vi "swabian_buffer_to_photons.vi"(0 "buffer":u64[](array[numeric]), 4 "Leftovers_in":T1, 5 "error in (no error)":errorcluster, 6 "sync_channel":i32, 8 "sync_period_ps":u64, 10 "first_batch":i32, 12 "first_sync_stamp":u64) -> (14 "output_buffer":u64[](array[numeric]), 15 "first_sync_stamp_out":u64, 18 "Leftovers_out":T1, 19 "error out":errorcluster)   [LabVIEW 2018]
uses:
  swabian_lib.dll
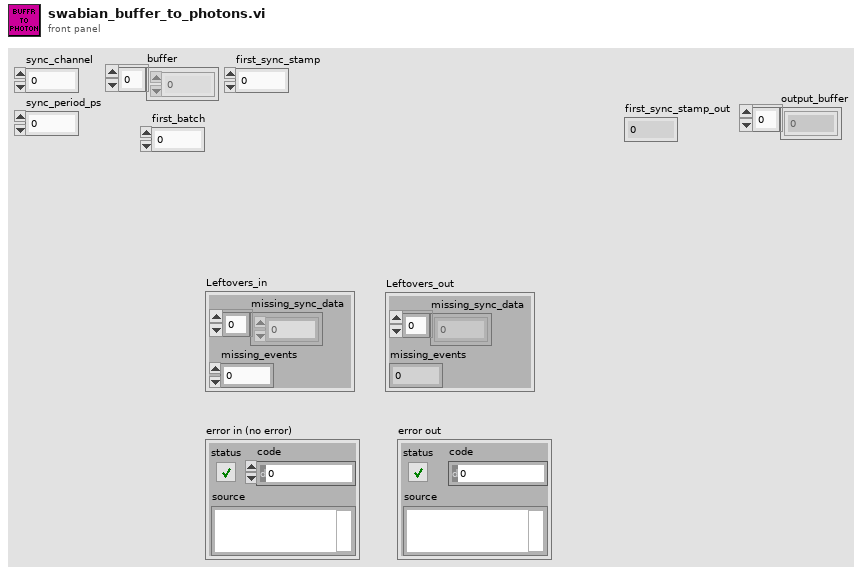
[diagram p1: front panel]
types:
  T1 = cluster{"missing_sync_data":u64[], "missing_events":i32}
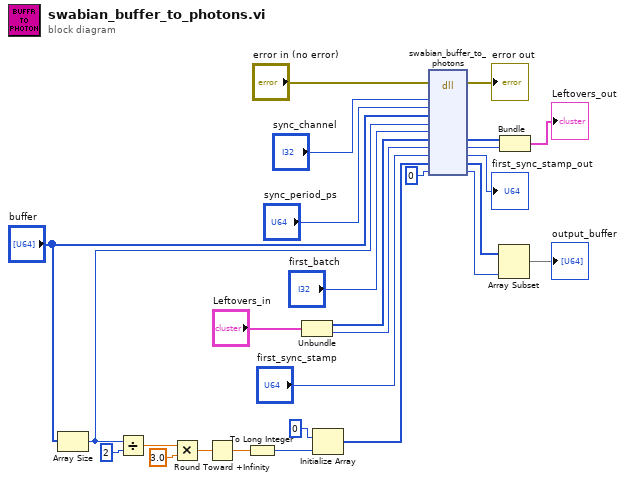
[diagram p0: block diagram]
diagram:
  n1 = Array Size(array="buffer") -> (size(s)=w18:i32)
  n2 = Divide(x=w18, y=2) -> (x/y=w16:dbl)
  n3 = Multiply(x=w16, y=3.0) -> (x*y=w14:dbl)
  n4 = Round Toward +Infinity(x=w14) -> (ceil(x): smallest int >= x=w13:dbl)
  n5 = To Long Integer(number=w13) -> (32bit integer=w12:i32)
  n6 = Unbundle("Leftovers_in") -> ("missing_sync_data"=w4:u64[], "missing_events"=w3:i32)
  n7 = Initialize Array(u64 0 ("element"), w12) -> (w11:u64[])
  n8 = dll-call lib="C:/Users/SWIR TCSPC/Desktop/Swabian/swabian_vis/swabian_lib/swabian_lib.dll" fn="swabian_buffer_to_photons"(error in="error in (no error)", "sync_channel"="sync_channel", "sync_period_ps"="sync_period_ps", "buffer"="buffer", "buffer_length"=w18, "first_batch"="first_batch", "missing_sync_data"=w4, "missing_events"=w3, "first_sync_stamp"="first_sync_stamp", "output_buffer"=w11, "output_length"=0) -> (error out=→"error out":errorcluster, "missing_sync_data"=w7:u64[], "missing_events"=w6:i32, "first_sync_stamp"=→"first_sync_stamp_out":u64, "output_buffer"=w10:u64[], "output_length"=w9:i32)  [unwired: 8 in, 1 out]
  n9 = Array Subset(array=w10, length=w9) -> (→"output_buffer":u64[])  [unwired: 1 in]
  n10 = Bundle("missing_sync_data"=w7, "missing_events"=w6) -> (→"Leftovers_out":T1)  [unwired: 1 in]
